vi "Log Application State.vi"(8 "error in (no error)":errorcluster, 11 "FSM State":T1) -> (0 "error out":errorcluster)   [LabVIEW 2017]
doc: "Logs the current application state to the system log."
uses:
  FSM States.ctl
  <vilib>/Utility/SystemLogging/NI_SystemLogging.lvlib
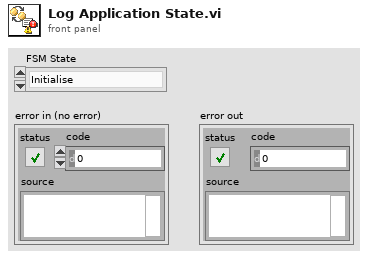
[diagram p1: front panel]
types:
  T1 = typedef "FSM States.ctl" = enum16{"Initialise", "Logging", "Close"}
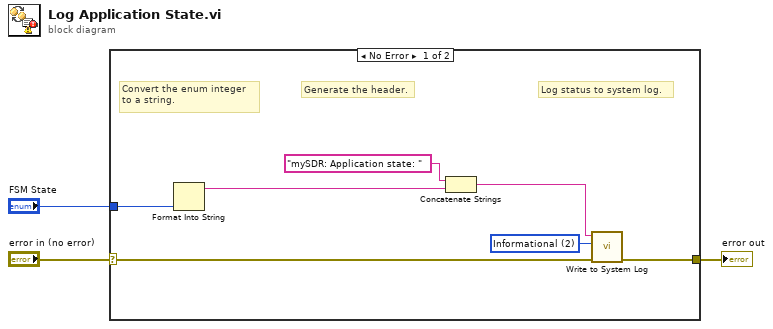
[diagram p0: block diagram]
diagram:
  n1 = case shown="No Error" "error in (no error)" {
    selector: "error in (no error)" -> [w4 w11]
    tunnel: [w8 w11] -> w3
    tunnel: "FSM State" -> [w5 _]
    frame No Error {
      w6 = 2 items=["Error", "Warning", "Informational"] ("severity")
      # "Convert the enum integer\nto a string."
      # "Generate the header."
      # "Log status to system log."
      n2 = Format Into String(w5) -> (resulting string=w10:string)  [unwired: 3 in, 1 out]
      n3 = Concatenate Strings("mySDR: Application state: ", w10) -> (w7:string)
      n4 = call <vilib>:"Write to System Log.vi"("error in (no error)"=w4, "severity"=w6, "message"=w7) -> ("error out"=w8:errorcluster)  [unwired: 8 in]
    }
    frame Error {
    }
  }
  "error out" <- w3
